vi "Set Multi.vi"(0 "Display State In":T1={"mixed"=FALSE, "format"="%#g", "Value"=0.0}, 7 "Value":dbl, 9 "Container State":T2, 11 "error in (no error)":errorcluster, 12 "First?":bool) -> (4 "Display State Out":T1={"mixed"=FALSE, "format"="%#g", "Value"=0.0}, 15 "error out":errorcluster)   [LabVIEW 2015, in "KNumeric (DBL).xctl"]
uses:
  KNumeric (DBL).xctl
  <vilib>/_xctls/Container State.ctl
  State.ctl
  <vilib>/_xctls/XControlSupport.lvlib
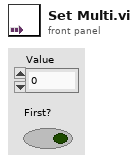
[diagram p1: front panel]
types:
  T1 = typedef "KNumeric (DBL).xctl/State.ctl" = cluster{"mixed":bool, "format":string, "Value":dbl}
  T2 = typedef "XControlSupport.lvlib/Container State.ctl" = cluster{"Indicator?":bool, "Run Mode?":bool, " Refnum":refnum<vi>}
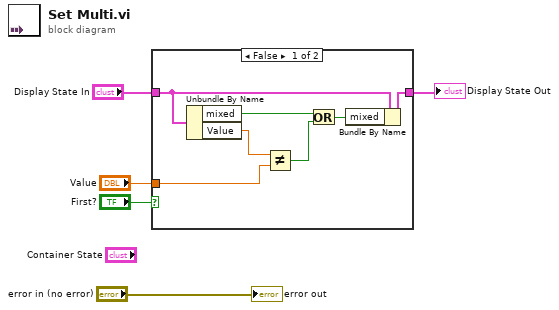
[diagram p0: block diagram]
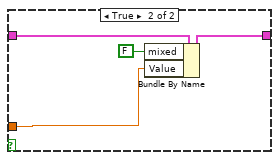
[diagram p2: hidden frame]
diagram:
  n1 = case shown="False" "First?" {
    tunnel: "Value" -> [w11 w13]
    tunnel: "Display State In" -> [w12 w16]
    tunnel: [w10 w15] -> w1
    frame False {
      n2 = Unbundle By Name(w12) -> ("mixed"=w8:bool, "Value"=w6:dbl)
      n3 = Not Equal?(x=w6, y=w11) -> (x != y?=w7:bool)
      n4 = Or(x=w8, y=w7) -> (x .or. y?=w9:bool)
      n5 = Bundle By Name(cluster=w12, "mixed"=w9) -> (w10:T1)
    }
    frame True {
      n6 = Bundle By Name(cluster=w16, "mixed"=FALSE ("Mixed value"), "Value"=w13) -> (w15:T1)
    }
  }
  "Display State Out" <- w1
  "error out" <- "error in (no error)"
